vi "Reset Device.vi"(0 "Session Handle in":T1, 11 "error in (no error)":errorcluster) -> (4 "Session Handle out":T1, 15 "error out":errorcluster)   [LabVIEW 2015, in "SLSC Switch.lvlib" / "SLSC Session.lvclass"]
uses:
  SLSC Session.lvclass
  Typedefs/Session Handle.ctl
  SLSC Session.lvclass/SLSC Session.ctl
  <vilib>/SLSC/SLSC.lvlib
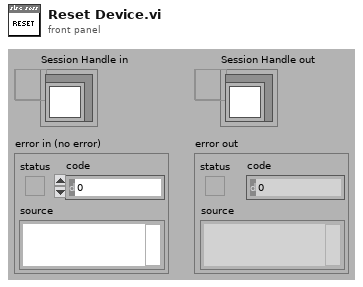
[diagram p1: front panel]
types:
  T1 = typedef "SLSC Switch.lvlib/SLSC Session.lvclass/Session Handle.ctl" = refnum<data-value>
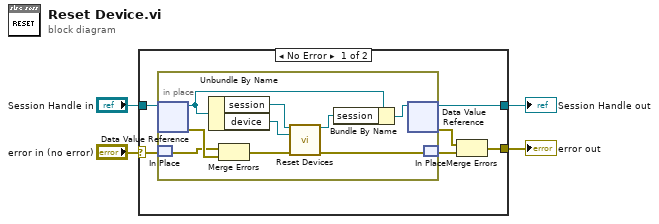
[diagram p0: block diagram]
diagram:
  n1 = case shown="No Error" "error in (no error)" {
    selector: "error in (no error)" -> [w5 w20]
    tunnel: "Session Handle in" -> [w10 w21]
    tunnel: [w9 w21] -> w3
    tunnel: [w6 w20] -> w2
    frame No Error {
      n2 = in-place {
        n3 = in-place-dvr #1(w10) -> (w13:refnum<class "SLSC Session.lvclass">, w19:errorcluster)
        n4 = in-place-match #2(w5) -> (w18:errorcluster)
        n5 = Unbundle By Name(w13) -> ("session"=w17:refnum<k21>, "device"=w16:refnum<k21>)
        n6 = Merge Errors(w18, w19) -> (w15:errorcluster)
        n7 = call <vilib>:"Reset Devices.vi"("session in"=w17, "devices"=w16, "error in (no error)"=w15) -> ("session out"=w12:refnum<k21>, "error out"=w14:errorcluster)  [unwired: 11 in]
        n8 = Bundle By Name(cluster=w13, "session"=w12) -> (w11:refnum<class "SLSC Session.lvclass">)
        n9 = in-place-dvr #1(w11) -> (w9:T1, w7:errorcluster)
        n10 = in-place-match #2(w14) -> (w8:errorcluster)
      }
      n11 = Merge Errors(w7, w8) -> (w6:errorcluster)
    }
    frame Error {
    }
  }
  "Session Handle out" <- w3
  "error out" <- w2
